vi "보안 시스템.vi"() -> ()   [LabVIEW 2018]
uses:
  <vilib>/Utility/file.llb/Write Delimited Spreadsheet (string).vi
panel:
  in  "시뮬레이션 중지":bool
  in  "영역 상태 알림":T1
  in  "탬퍼 스위치":cluster{bool, bool, bool, bool, bool, bool}
  in  "바이패스 스위치":cluster{bool, bool, bool, bool, bool, bool}
  in  "알람 스위치":cluster{bool, bool, bool, bool, bool, bool}
  # "초록색 : 정상\n 빨간색 : 알람\n 파란색 : 바이패스\n 주황색 : 탬퍼"
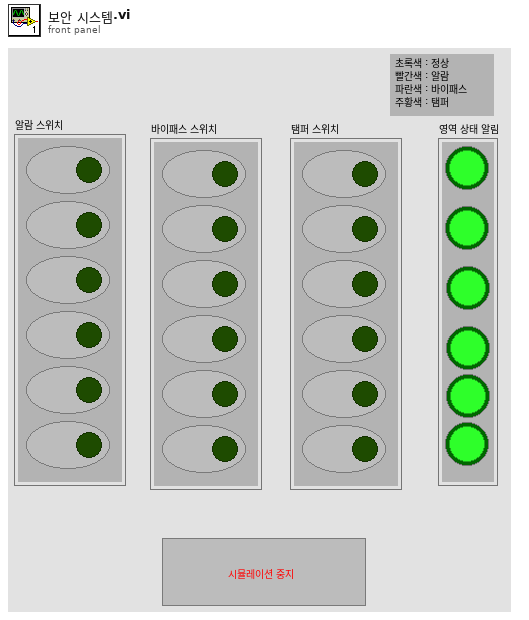
[diagram p1: front panel]
types:
  T1 = cluster{"1":bool, "2":bool, "3":bool, "4":bool, "5":bool, "6":bool}
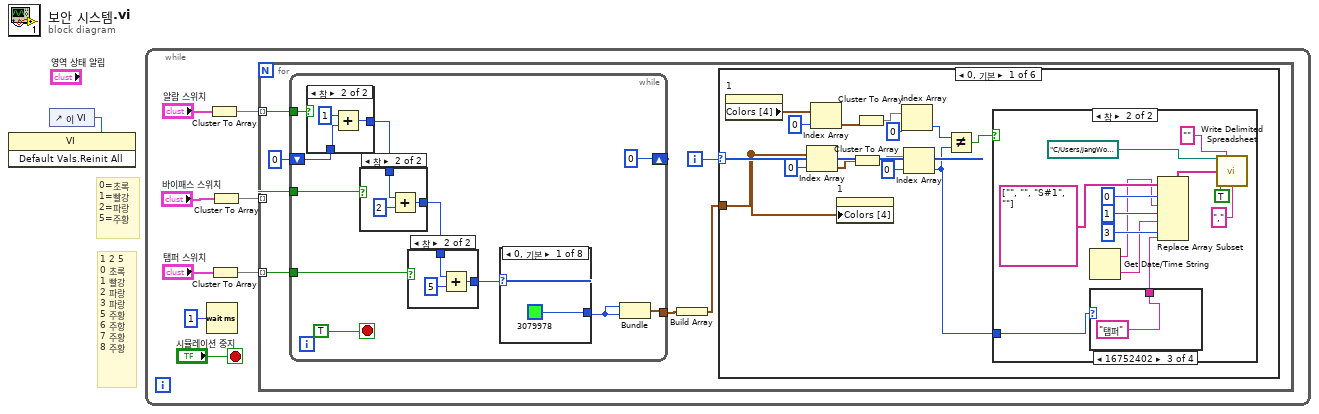
[diagram p0: block diagram]
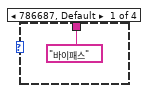
[diagram p3: hidden frame]
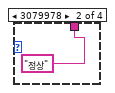
[diagram p4: hidden frame]
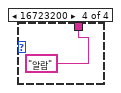
[diagram p5: hidden frame]
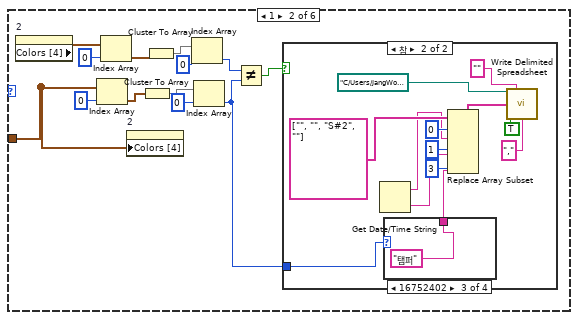
[diagram p6: hidden frame]
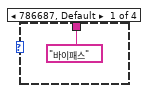
[diagram p8: hidden frame]
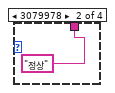
[diagram p9: hidden frame]
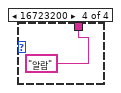
[diagram p10: hidden frame]
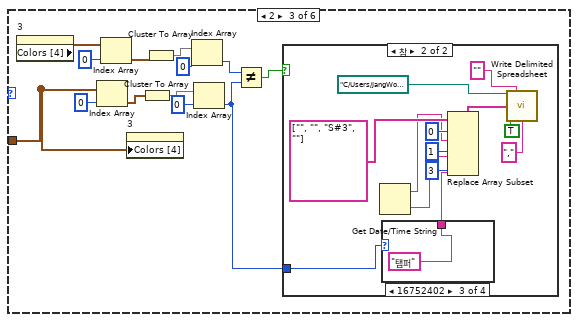
[diagram p11: hidden frame]
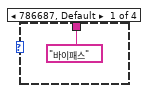
[diagram p13: hidden frame]
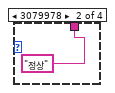
[diagram p14: hidden frame]
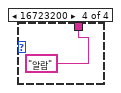
[diagram p15: hidden frame]
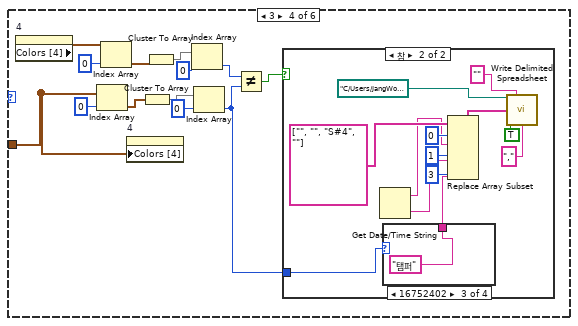
[diagram p16: hidden frame]
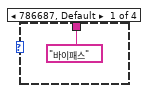
[diagram p18: hidden frame]
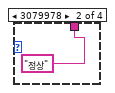
[diagram p19: hidden frame]
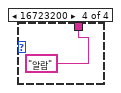
[diagram p20: hidden frame]
diagram:
  # "1 2 5\n0 초록\n1 빨강\n2 파랑\n3 파랑\n5 주황\n6 주항\n7 주황\n8 주황"
  # "0=초록\n1=빨강\n2=파랑\n5=주황"
  n1 = control-ref of="이 VI"() -> (w1:refnum<vi>)
  n2 = invoke class="VI" method="Default Vals.Reinit All"(reference=w1) -> ()  [unwired: 2 in, 3 out]
  n3 = while {
    stop <- "시뮬레이션 중지" stop-if-true
    n4 = Wait (ms)(milliseconds to wait=u32 1 ("대기 시간 (ms)")) -> ()  [unwired: 1 out]
    n5 = Cluster To Array(cluster="알람 스위치") -> (array=w8:bool[])
    n6 = Cluster To Array(cluster="탬퍼 스위치") -> (array=w4:bool[])
    n7 = Cluster To Array(cluster="바이패스 스위치") -> (array=w6:bool[])
    n8 = for {
      tunnel: w8 -> [w15] mode=indexing
      tunnel: w6 -> [w14] mode=indexing
      tunnel: w4 -> [w13] mode=indexing
      i -> [w10]
      n9 = while {
        shift-right: [0] -> _
        shift-left: 0 -> [w202]
        tunnel: w15 -> [w201]
        tunnel: w14 -> [w200]
        tunnel: w13 -> [w199]
        tunnel: [w197] -> w12
        stop <- TRUE stop-if-true
        n10 = case shown="참" w201 {
          tunnel: w202 -> [w216 w219]
          tunnel: [w216 w217] -> w207
          frame False {
          }
          frame True {
            n11 = Add(x=1, y=w219) -> (x+y=w217:i32)
          }
        }
        n12 = case shown="참" w200 {
          tunnel: w207 -> [w212 w215]
          tunnel: [w212 w214] -> w206
          frame False {
          }
          frame True {
            n13 = Add(x=w215, y=2) -> (x+y=w214:i32)
          }
        }
        n14 = case shown="참" w199 {
          tunnel: w206 -> [w208 w211]
          tunnel: [w208 w210] -> w204
          frame False {
          }
          frame True {
            n15 = Add(x=w211, y=5) -> (x+y=w210:i32)
          }
        }
        n16 = case shown="0, 기본" w204 {
          tunnel: [u32 3079978 u32 16723200 u32 786687 u32 786687 u32 16752402 u32 16752402 u32 16752402 u32 16752402] -> w205
          frame 0, Default {
          }
          frame 1 {
          }
          frame 2 {
          }
          frame 3 {
          }
          frame 5 {
          }
          frame 6 {
          }
          frame 7 {
          }
          frame 8 {
          }
        }
        n17 = Bundle(w205, w205) -> (w197:cluster{u32, u32})  [unwired: 1 in]
      }
      n18 = Build Array(w12) -> (w11:cluster{u32, u32}[])
      n19 = case shown="0, 기본" w10 {
        tunnel: w11 -> [w26 w56 w86 w116 w146 w176]
        frame 0, Default {
          n20 = property on="1" class="Bool (엄격한)"() -> ("Colors [4]"=w28:cluster{u32, u32}[])  [unwired: 2 in, 2 out]
          n21 = Index Array(array=w26, index=0 ("인덱스")) -> (element=w22:cluster{u32, u32})
          n22 = Index Array(array=w28, index=0 ("인덱스")) -> (element=w25:cluster{u32, u32})
          n23 = property on="1" class="Bool (엄격한)"("Colors [4]"=w26) -> ()  [unwired: 2 in, 2 out]
          n24 = Cluster To Array(cluster=w22) -> (array=w21:u32[])
          n25 = Cluster To Array(cluster=w25) -> (array=w24:u32[])
          n26 = Index Array(array=w24, index=0 ("인덱스")) -> (element=w19:u32)
          n27 = Index Array(array=w21, index=0 ("인덱스")) -> (element=w17:u32)
          n28 = Not Equal?(x=w19, y=w17) -> (x != y?=w18:bool)
          n29 = case shown="참" w18 {
            tunnel: w17 -> [_ w31]
            frame False {
            }
            frame True {
              n30 = Get Date/Time String() -> (date string=w33:string, time string=w32:string)  [unwired: 3 in]
              n31 = case shown="16752402" w31 {
                tunnel: ["바이패스" "정상" "탬퍼" "알람"] -> w30
                frame 786687, Default {
                }
                frame 3079978 {
                }
                frame 16752402 {
                }
                frame 16723200 {
                }
              }
              n32 = Replace Array Subset(array=string[] ["", "", "S#1", ""], new element #1=w33, index #1=0 ("인덱스"), new element #2=w32, index #2=1 ("인덱스"), new element #3=w30, index #3=3 ("인덱스")) -> (w38:string[])
              n33 = call-poly <vilib>:"Write Delimited Spreadsheet.vi"("file path (dialog if empty)"=path "C:/Users/JangWoo/Documents/labview study/test.csv", "format (%s)"="", "1D data"=w38, "append to file? (new file:F)"=TRUE, "delimiter (\\t)"="," ("delimiter (\\t)")) -> ()  [unwired: 9 in, 2 out]
            }
          }
        }
        frame 1 {
          n34 = property on="2" class="Bool (엄격한)"() -> ("Colors [4]"=w58:cluster{u32, u32}[])  [unwired: 2 in, 2 out]
          n35 = Index Array(array=w56, index=0 ("인덱스")) -> (element=w52:cluster{u32, u32})
          n36 = Index Array(array=w58, index=0 ("인덱스")) -> (element=w55:cluster{u32, u32})
          n37 = property on="2" class="Bool (엄격한)"("Colors [4]"=w56) -> ()  [unwired: 2 in, 2 out]
          n38 = Cluster To Array(cluster=w52) -> (array=w51:u32[])
          n39 = Cluster To Array(cluster=w55) -> (array=w54:u32[])
          n40 = Index Array(array=w54, index=0 ("인덱스")) -> (element=w49:u32)
          n41 = Index Array(array=w51, index=0 ("인덱스")) -> (element=w47:u32)
          n42 = Not Equal?(x=w49, y=w47) -> (x != y?=w48:bool)
          n43 = case shown="참" w48 {
            tunnel: w47 -> [_ w61]
            frame False {
            }
            frame True {
              n44 = Get Date/Time String() -> (date string=w63:string, time string=w62:string)  [unwired: 3 in]
              n45 = case shown="16752402" w61 {
                tunnel: ["바이패스" "정상" "탬퍼" "알람"] -> w60
                frame 786687, Default {
                }
                frame 3079978 {
                }
                frame 16752402 {
                }
                frame 16723200 {
                }
              }
              n46 = Replace Array Subset(array=string[] ["", "", "S#2", ""], new element #1=w63, index #1=0 ("인덱스"), new element #2=w62, index #2=1 ("인덱스"), new element #3=w60, index #3=3 ("인덱스")) -> (w68:string[])
              n47 = call-poly <vilib>:"Write Delimited Spreadsheet.vi"("file path (dialog if empty)"=path "C:/Users/JangWoo/Documents/labview study/test.csv", "format (%s)"="", "1D data"=w68, "append to file? (new file:F)"=TRUE, "delimiter (\\t)"="," ("delimiter (\\t)")) -> ()  [unwired: 9 in, 2 out]
            }
          }
        }
        frame 2 {
          n48 = property on="3" class="Bool (엄격한)"() -> ("Colors [4]"=w88:cluster{u32, u32}[])  [unwired: 2 in, 2 out]
          n49 = Index Array(array=w86, index=0 ("인덱스")) -> (element=w82:cluster{u32, u32})
          n50 = Index Array(array=w88, index=0 ("인덱스")) -> (element=w85:cluster{u32, u32})
          n51 = property on="3" class="Bool (엄격한)"("Colors [4]"=w86) -> ()  [unwired: 2 in, 2 out]
          n52 = Cluster To Array(cluster=w82) -> (array=w81:u32[])
          n53 = Cluster To Array(cluster=w85) -> (array=w84:u32[])
          n54 = Index Array(array=w84, index=0 ("인덱스")) -> (element=w79:u32)
          n55 = Index Array(array=w81, index=0 ("인덱스")) -> (element=w77:u32)
          n56 = Not Equal?(x=w79, y=w77) -> (x != y?=w78:bool)
          n57 = case shown="참" w78 {
            tunnel: w77 -> [_ w91]
            frame False {
            }
            frame True {
              n58 = Get Date/Time String() -> (date string=w93:string, time string=w92:string)  [unwired: 3 in]
              n59 = case shown="16752402" w91 {
                tunnel: ["바이패스" "정상" "탬퍼" "알람"] -> w90
                frame 786687, Default {
                }
                frame 3079978 {
                }
                frame 16752402 {
                }
                frame 16723200 {
                }
              }
              n60 = Replace Array Subset(array=string[] ["", "", "S#3", ""], new element #1=w93, index #1=0 ("인덱스"), new element #2=w92, index #2=1 ("인덱스"), new element #3=w90, index #3=3 ("인덱스")) -> (w98:string[])
              n61 = call-poly <vilib>:"Write Delimited Spreadsheet.vi"("file path (dialog if empty)"=path "C:/Users/JangWoo/Documents/labview study/test.csv", "format (%s)"="", "1D data"=w98, "append to file? (new file:F)"=TRUE, "delimiter (\\t)"="," ("delimiter (\\t)")) -> ()  [unwired: 9 in, 2 out]
            }
          }
        }
        frame 3 {
          n62 = property on="4" class="Bool (엄격한)"() -> ("Colors [4]"=w118:cluster{u32, u32}[])  [unwired: 2 in, 2 out]
          n63 = Index Array(array=w116, index=0 ("인덱스")) -> (element=w112:cluster{u32, u32})
          n64 = Index Array(array=w118, index=0 ("인덱스")) -> (element=w115:cluster{u32, u32})
          n65 = property on="4" class="Bool (엄격한)"("Colors [4]"=w116) -> ()  [unwired: 2 in, 2 out]
          n66 = Cluster To Array(cluster=w112) -> (array=w111:u32[])
          n67 = Cluster To Array(cluster=w115) -> (array=w114:u32[])
          n68 = Index Array(array=w114, index=0 ("인덱스")) -> (element=w109:u32)
          n69 = Index Array(array=w111, index=0 ("인덱스")) -> (element=w107:u32)
          n70 = Not Equal?(x=w109, y=w107) -> (x != y?=w108:bool)
          n71 = case shown="참" w108 {
            tunnel: w107 -> [_ w121]
            frame False {
            }
            frame True {
              n72 = Get Date/Time String() -> (date string=w123:string, time string=w122:string)  [unwired: 3 in]
              n73 = case shown="16752402" w121 {
                tunnel: ["바이패스" "정상" "탬퍼" "알람"] -> w120
                frame 786687, Default {
                }
                frame 3079978 {
                }
                frame 16752402 {
                }
                frame 16723200 {
                }
              }
              n74 = Replace Array Subset(array=string[] ["", "", "S#4", ""], new element #1=w123, index #1=0 ("인덱스"), new element #2=w122, index #2=1 ("인덱스"), new element #3=w120, index #3=3 ("인덱스")) -> (w128:string[])
              n75 = call-poly <vilib>:"Write Delimited Spreadsheet.vi"("file path (dialog if empty)"=path "C:/Users/JangWoo/Documents/labview study/test.csv", "format (%s)"="", "1D data"=w128, "append to file? (new file:F)"=TRUE, "delimiter (\\t)"="," ("delimiter (\\t)")) -> ()  [unwired: 9 in, 2 out]
            }
          }
        }
        frame 4 {
          n76 = property on="5" class="Bool (엄격한)"() -> ("Colors [4]"=w148:cluster{u32, u32}[])  [unwired: 2 in, 2 out]
          n77 = Index Array(array=w146, index=0 ("인덱스")) -> (element=w142:cluster{u32, u32})
          n78 = Index Array(array=w148, index=0 ("인덱스")) -> (element=w145:cluster{u32, u32})
          n79 = property on="5" class="Bool (엄격한)"("Colors [4]"=w146) -> ()  [unwired: 2 in, 2 out]
          n80 = Cluster To Array(cluster=w142) -> (array=w141:u32[])
          n81 = Cluster To Array(cluster=w145) -> (array=w144:u32[])
          n82 = Index Array(array=w144, index=0 ("인덱스")) -> (element=w139:u32)
          n83 = Index Array(array=w141, index=0 ("인덱스")) -> (element=w137:u32)
          n84 = Not Equal?(x=w139, y=w137) -> (x != y?=w138:bool)
          n85 = case shown="참" w138 {
            tunnel: w137 -> [_ w151]
            frame False {
            }
            frame True {
              n86 = Get Date/Time String() -> (date string=w153:string, time string=w152:string)  [unwired: 3 in]
              n87 = case shown="16752402" w151 {
                tunnel: ["바이패스" "정상" "탬퍼" "알람"] -> w150
                frame 786687, Default {
                }
                frame 3079978 {
                }
                frame 16752402 {
                }
                frame 16723200 {
                }
              }
              n88 = Replace Array Subset(array=string[] ["", "", "S#5", ""], new element #1=w153, index #1=0 ("인덱스"), new element #2=w152, index #2=1 ("인덱스"), new element #3=w150, index #3=3 ("인덱스")) -> (w158:string[])
              n89 = call-poly <vilib>:"Write Delimited Spreadsheet.vi"("file path (dialog if empty)"=path "C:/Users/JangWoo/Documents/labview study/test.csv", "format (%s)"="", "1D data"=w158, "append to file? (new file:F)"=TRUE, "delimiter (\\t)"="," ("delimiter (\\t)")) -> ()  [unwired: 9 in, 2 out]
            }
          }
        }
        frame 5 {
          n90 = property on="6" class="Bool (엄격한)"() -> ("Colors [4]"=w178:cluster{u32, u32}[])  [unwired: 2 in, 2 out]
          n91 = Index Array(array=w176, index=0 ("인덱스")) -> (element=w172:cluster{u32, u32})
          n92 = Index Array(array=w178, index=0 ("인덱스")) -> (element=w175:cluster{u32, u32})
          n93 = property on="6" class="Bool (엄격한)"("Colors [4]"=w176) -> ()  [unwired: 2 in, 2 out]
          n94 = Cluster To Array(cluster=w172) -> (array=w171:u32[])
          n95 = Cluster To Array(cluster=w175) -> (array=w174:u32[])
          n96 = Index Array(array=w174, index=0 ("인덱스")) -> (element=w169:u32)
          n97 = Index Array(array=w171, index=0 ("인덱스")) -> (element=w167:u32)
          n98 = Not Equal?(x=w169, y=w167) -> (x != y?=w168:bool)
          n99 = case shown="참" w168 {
            tunnel: w167 -> [_ w181]
            frame False {
            }
            frame True {
              n100 = Get Date/Time String() -> (date string=w183:string, time string=w182:string)  [unwired: 3 in]
              n101 = case shown="16752402" w181 {
                tunnel: ["바이패스" "정상" "탬퍼" "알람"] -> w180
                frame 786687, Default {
                }
                frame 3079978 {
                }
                frame 16752402 {
                }
                frame 16723200 {
                }
              }
              n102 = Replace Array Subset(array=string[] ["", "", "S#6", ""], new element #1=w183, index #1=0 ("인덱스"), new element #2=w182, index #2=1 ("인덱스"), new element #3=w180, index #3=3 ("인덱스")) -> (w188:string[])
              n103 = call-poly <vilib>:"Write Delimited Spreadsheet.vi"("file path (dialog if empty)"=path "C:/Users/JangWoo/Documents/labview study/test.csv", "format (%s)"="", "1D data"=w188, "append to file? (new file:F)"=TRUE, "delimiter (\\t)"="," ("delimiter (\\t)")) -> ()  [unwired: 9 in, 2 out]
            }
          }
        }
      }
    }
  }
